vi "close connhandler pool.vi"(8 "error in (no error)":errorcluster, 11 "VI ref":variant) -> (0 "error out":errorcluster)   [LabVIEW 2015]
uses:
  TCP connection/TCP connection.lvclass
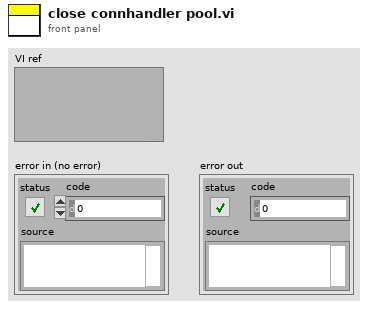
[diagram p1: front panel]
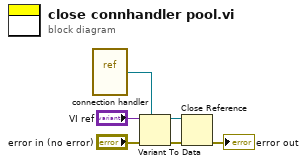
[diagram p0: block diagram]
diagram:
  n1 = vi-ref "connection handler.vi"() -> (w6:refnum<vi>)
  n2 = Variant To Data(error in="error in (no error)", type=w6, Variant="VI ref") -> (data=w4:refnum<vi>, error out=w3:errorcluster)
  n3 = Close Reference(reference=w4, error in (no error)=w3) -> (error out=→"error out":errorcluster)
